vi "Initialise.vi"(6 "Name":string, 9 "Metadata":string, 10 "Enabled (T)":bool=TRUE, 11 "Period [s]":dbl) -> (3 "Timer out":refnum<class "Timer.lvclass">)   [LabVIEW 2015, in "Timer.lvclass"]
uses:
  Timer.lvclass
  Timer.lvclass/Timer.ctl
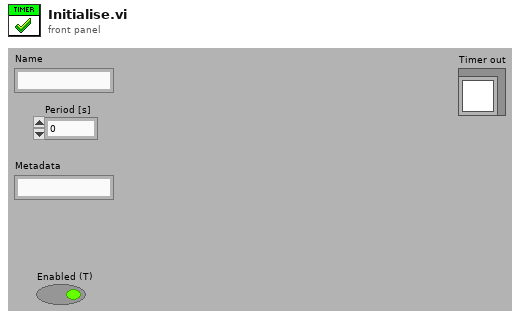
[diagram p1: front panel]
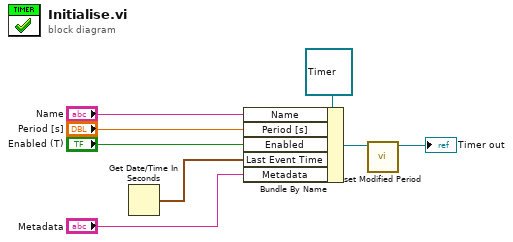
[diagram p0: block diagram]
diagram:
  n1 = Get Date/Time In Seconds() -> (seconds since 1Jan1904=w5:timestamp)
  n2 = Bundle By Name(cluster=refnum<class "Timer.lvclass"> refnum ("Event.lvclass"), "Name"="Name", "Period [s]"="Period [s]", "Enabled"="Enabled (T)", "Last Event Time"=w5, "Metadata"="Metadata") -> (w2:refnum<class "Timer.lvclass">)
  n3 = call "set Modified Period.vi"("Timer in"=w2) -> ("Timer out"=→"Timer out":refnum<class "Timer.lvclass">)  [unwired: 10 in]
